vi "SoftwarePhase.vi"() -> ()   [LabVIEW 2012]
uses:
  <vilib>/imath/engines/lvmath/Plug In/_Char/NIMS_CH_character datatype.ctl
  <vilib>/Utility/inputDevices.llb/closeKeyboard.vi
  <vilib>/imath/engines/lvmath2/RunTimeEngine/ErrorHandling/NIMS_Finalize Error.vi
  <vilib>/imath/engines/lvmath2/RunTimeEngine/Managers/WorkSpace/UID Generator.vi
  <vilib>/imath/engines/lvmath2/RunTimeEngine/Managers/SymbolTable/Clear UID.vi
  <vilib>/imath/engines/lvmath/Plug In/_Char/NIMS_CH_Character RV to String.vi
  <vilib>/imath/engines/lvmath2/RunTimeEngine/NodeEndStatement/NIMS_NodeEndStatement_Output.vi
  <instcachedir>/0/NIMS_NodeEndStatement_Output_53EC0D466D134D7ABD903AC30B43404B.lvgen/NIMS_NodeEndStatement_Output_53EC0D466D134D7ABD903AC30B43404B_009.vi
  <vilib>/imath/engines/lvmath2/RunTimeEngine/RunTimeType/NIMS_RunTimeType_From StrictType (excl LVString).vi
  <instcachedir>/0/NIMS_RunTimeType_From StrictType (excl LVString)_AC52D965D0864706932D20A05968E122.lvgen/NIMS_RunTimeType_From StrictType (excl LVString)_AC52D965D0864706932D20A05968E122_001.vi
  <vilib>/imath/engines/lvmath2/RunTimeEngine/LocalVariableDefStatement/MC_LocalVariableDefStatement_Display.vi
  <vilib>/imath/engines/lvmath2/RunTimeEngine/VariableToken/NIMS_VariableToken_CondDefined.vi
  <instcachedir>/0/NIMS_VariableToken_CondDefined_295AAB8C64C949DA8EA45AB7820AF759.lvgen/NIMS_VariableToken_CondDefined_295AAB8C64C949DA8EA45AB7820AF759_004.vi
  <vilib>/imathl/engines/lvmath/Functions/Error Handling/Create Error.vi
  <instcachedir>/0/NIMS_NodeEndStatement_Output_53EC0D466D134D7ABD903AC30B43404B.lvgen/NIMS_NodeEndStatement_Output_53EC0D466D134D7ABD903AC30B43404B_012.vi
  <instcachedir>/0/NIMS_RunTimeType_From StrictType (excl LVString)_AC52D965D0864706932D20A05968E122.lvgen/NIMS_RunTimeType_From StrictType (excl LVString)_AC52D965D0864706932D20A05968E122_000.vi
  <vilib>/imath/engines/lvmath2/RunTimeEngine/RunTimeType/NIMS_RunTimeType_Set Source Original Bool.vi
  <vilib>/Utility/inputDevices.llb/keyboardAcquire.vi
  <instcachedir>/0/NIMS_NodeEndStatement_Output_53EC0D466D134D7ABD903AC30B43404B.lvgen/NIMS_NodeEndStatement_Output_53EC0D466D134D7ABD903AC30B43404B_010.vi
  <vilib>/imath/engines/lvmath2/RunTimeEngine/Managers/SymbolTable/NIMS_WorkSpace.lvlib
panel:
  out "Simulation UDP":bool
  out "BS Timed Out":bool
  out "Base Station":string
  in  "error in (no error)":errorcluster
  in  "Tab Control":T1(tab)
  out "Bump Sensor 2":bool
  out "Distance 2, CM":dbl
  out "IR Volts 2":dbl
  out "Red":dbl(knob) scale=0.0..100.0
  out "Green":dbl(knob) scale=0.0..100.0
  out "Blue":dbl(knob) scale=0.0..100.0
  out "Color Chosen":u32(colorbox)
  out "Bump Sensor 1":bool
  out "IR Volts 1":dbl
  out "Distance 1, CM":dbl
  in  "stop":bool
  out "Left Rudder":i32
  out "Right Rudder":i32
  in  "Rudders":i32(slide)=1500 scale=500.0..2500.0
  out "Port\nMotor":i32
  out "Starboard\nMotor":i32
  out "Port Speed":i32(knob) scale=1000.0..2000.0
  out "Starboard Speed":i32(knob) scale=1000.0..2000.0
  in  "Pan Camera":i32(slide)=1500 scale=500.0..2500.0
  out "Speed Balance":i32(knob) scale=-600.0..600.0
  out "Angle to Target":i32
  out "Distance to Target":i32
  out "IR 2":bool
  out "IR 1":bool
  out "Bump 2":bool
  out "Bump  1":bool
  out "Current Target":i32
  out "Obstacle Detected":bool
  out "Primitive Engaged":string
  out "Desired Heading":i32
  out "Target Y":i32
  out "Target X":i32
  out "Current Y":i32
  out "Current X":i32
  out "Current Heading":i32
  in  "Target Approaching":i32
  out "Target Locations":i32[][](array[numeric])
  in  "Step Size":i32=5
  in  "PC Status":i32=1
  out "String Received":string
  out "return count":u32
  out "bytes written":u32
  out "Blinky":bool
  in  "String":string="$CS1500P1500R1500L1500P1500H   1\n"
  in  "FULLSTOP":bool
  in  "VISA resource name":refnum<visa-resource-name>="COM7"
  # "ROBOT CONTROL VI\nSoftware Phase for Autonomy\n\nVPreston\n3/20/2014"
  # "Use this tab to make sure your sensors are happy and working properly."
  # "Motor Control"
  # "Direction of thrust"
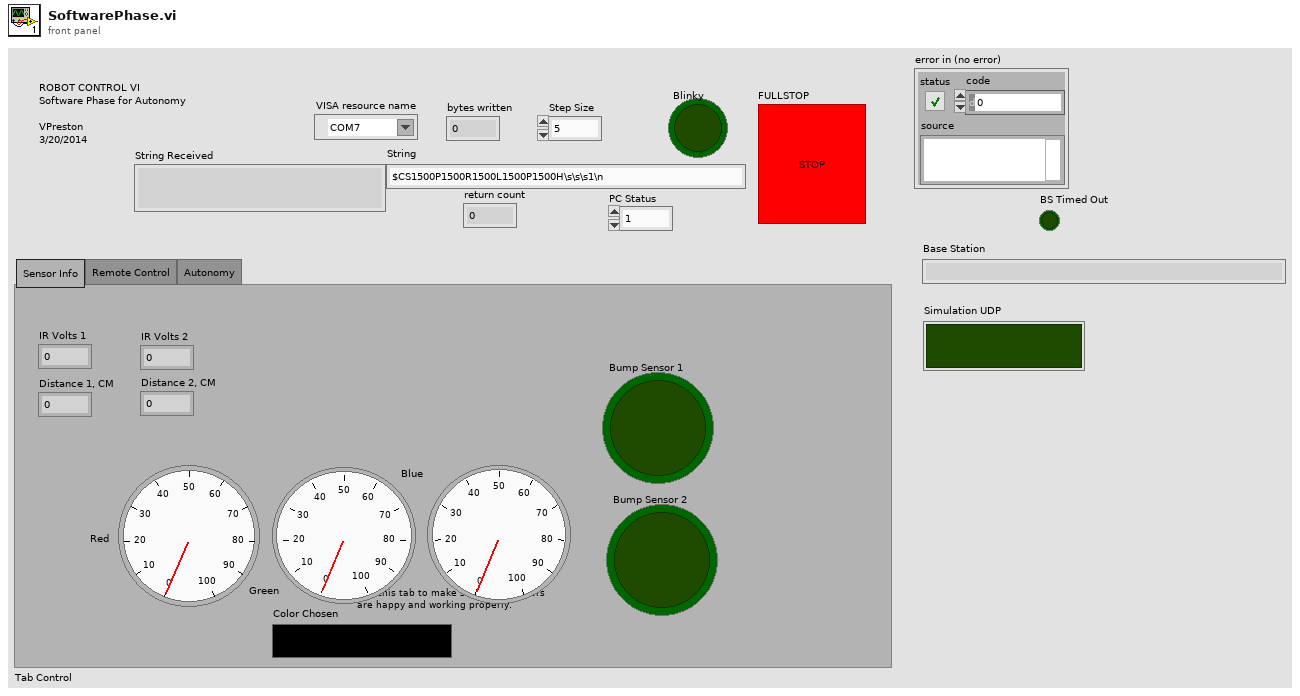
[diagram p1: front panel]
types:
  T1 = enum32{"Sensor Info", "Remote Control", "Autonomy"}
  T2 = enum16{"0", "1", "2", "3", "4", "5", "6", "7", "8", "9", "A", "B", "C", "D", "E", "F", "G", "H", "I", "J", "K", "L", "M", "N", "O", "P", "Q", "R", "S", "T", "U", "V", "W", "X", "Y", "Z", "F1", "F2", "F3", "F4", "F5", "F6", "F7", "F8", "F9", "F10", "F11", "F12", "F13", "F14", "F15", "ADD", "BACK", "BACKSLASH", "CAPITAL", "COMMA", "DECIMAL", "DELETE", "DIVIDE", "DOWN", "END", "EQUALS", "ESCAPE", "GRAVE (`)", "HOME", "INSERT", "LBRACKET", "LCONTROL", "LEFT", "L ALT", "LSHIFT", "LWIN", "MINUS", "MULTIPLY", "NEXT", "NUMLOCK", "NUMPAD_0", "NUMPAD_1", "NUMPAD_2", "NUMPAD_3", "NUMPAD_4", "NUMPAD_5", "NUMPAD_6", "NUMPAD_7", "NUMPAD_8", "NUMPAD_9", "PAUSE", "PERIOD", "PRIOR (PG UP)", "RBRACKET", "RCONTROL", "RETURN", "RIGHT", "R ALT", "RSHIFT", "RWIN", "SCROLL", "SEMICOLON", "SLASH", "SPACE", "SUBTRACT", "TAB", "UP", "ENTER (num pad)", "' (quote)"}[]
  T3 = enum16{"0", "1", "2", "3", "4", "5", "6", "7", "8", "9", "A", "B", "C", "D", "E", "F", "G", "H", "I", "J", "K", "L", "M", "N", "O", "P", "Q", "R", "S", "T", "U", "V", "W", "X", "Y", "Z", "F1", "F2", "F3", "F4", "F5", "F6", "F7", "F8", "F9", "F10", "F11", "F12", "F13", "F14", "F15", "ADD", "BACK", "BACKSLASH", "CAPITAL", "COMMA", "DECIMAL", "DELETE", "DIVIDE", "DOWN", "END", "EQUALS", "ESCAPE", "GRAVE (`)", "HOME", "INSERT", "LBRACKET", "LCONTROL", "LEFT", "L ALT", "LSHIFT", "LWIN", "MINUS", "MULTIPLY", "NEXT", "NUMLOCK", "NUMPAD_0", "NUMPAD_1", "NUMPAD_2", "NUMPAD_3", "NUMPAD_4", "NUMPAD_5", "NUMPAD_6", "NUMPAD_7", "NUMPAD_8", "NUMPAD_9", "PAUSE", "PERIOD", "PRIOR (PG UP)", "RBRACKET", "RCONTROL", "RETURN", "RIGHT", "R ALT", "RSHIFT", "RWIN", "SCROLL", "SEMICOLON", "SLASH", "SPACE", "SUBTRACT", "TAB", "UP", "ENTER (num pad)", "' (quote)"}
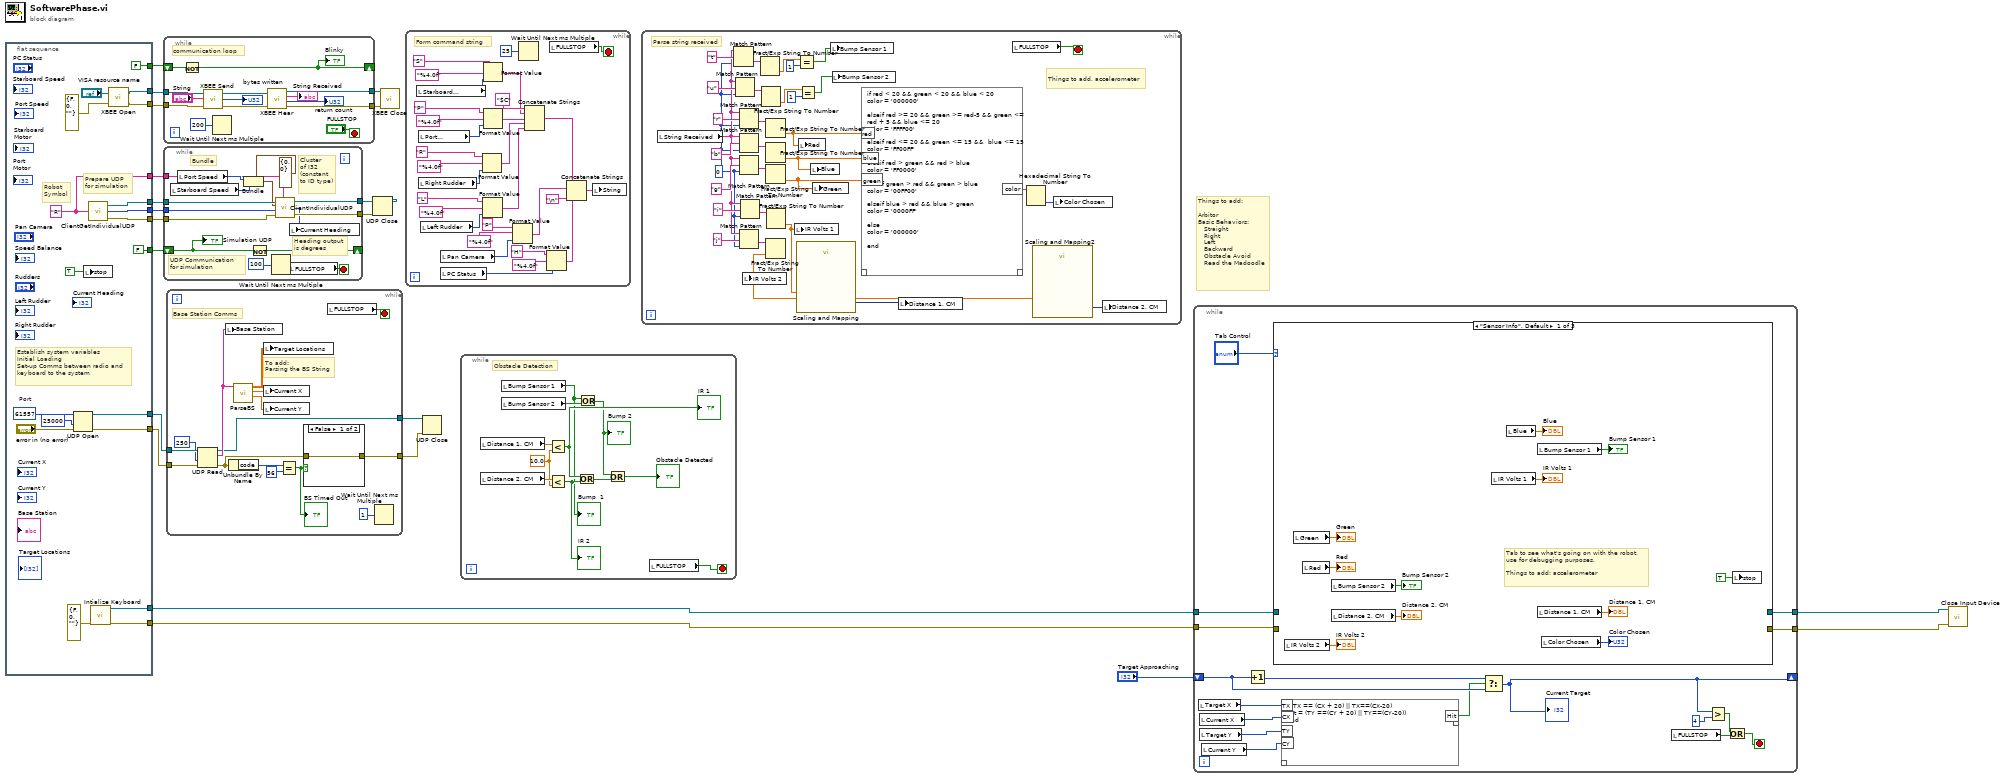
[diagram p0: block diagram]
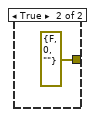
[diagram p2: hidden frame]
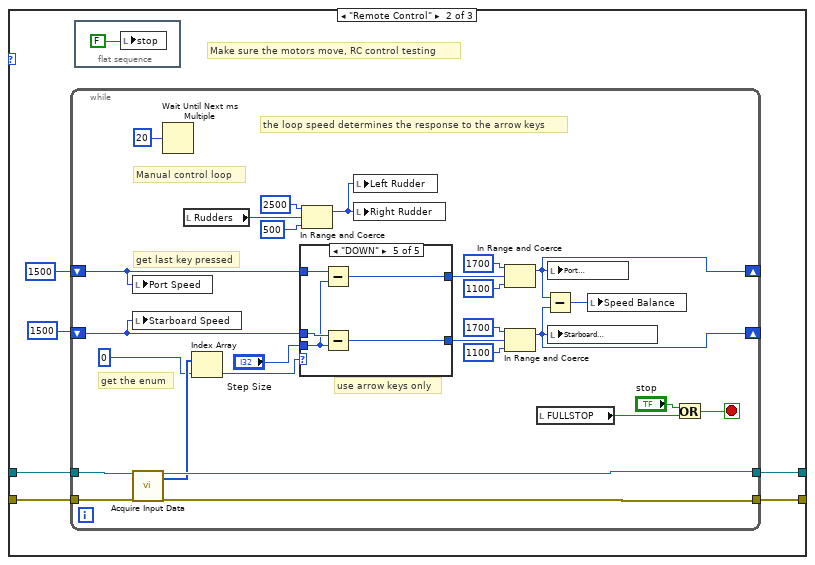
[diagram p3: hidden frame]
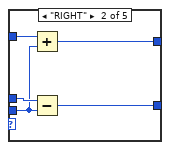
[diagram p5: hidden frame]
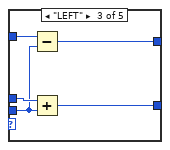
[diagram p6: hidden frame]
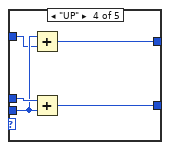
[diagram p7: hidden frame]
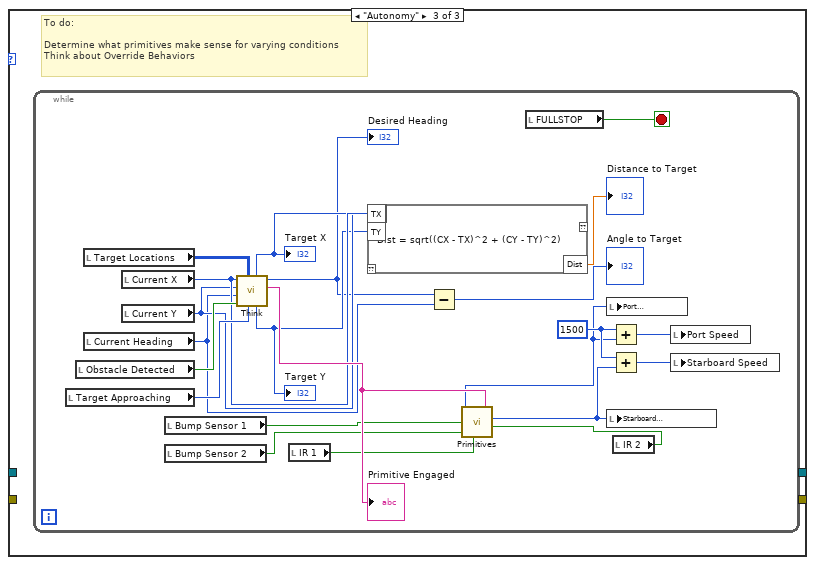
[diagram p8: hidden frame]
diagram:
  # "Things to add: \n\nArbitor\nBasic Behaviors:\n   Straight\n   Right\n   Left\n   Backward\n   Obstacle Avoid\n   Read the Madoodle"
  n1 = flat-sequence {
    tunnel: [w40] -> w21
    tunnel: [w23] -> w20
    tunnel: [FALSE] -> w17
    tunnel: [w35] -> w16
    tunnel: [w34] -> w15
    tunnel: [w29] -> w8
    tunnel: [w28] -> w12
    tunnel: [w27] -> w7
    tunnel: [w26] -> w5
    tunnel: [w25] -> w6
    tunnel: [w24] -> w4
    tunnel: [FALSE] -> w1
    frame #0 {
      w24 = "R"
      w31 = u16 61557  # Port
      # "Prepare UDP\nfor simulation"
      # "Robot \nSymbol"
      # "Establish system variables\nInitial Loading\nSet-up Comms between radio and\nkeyboard to the system"
      n2 = UDP Open(8:"error in (no error)", 9:25000 ("timeout ms (25000)"), 11:w31) -> (port=w29:refnum<k16>, 0:w28:errorcluster)  [unwired: 2 in, 1 out]
      n3 = local write "stop"(TRUE) -> ()
      n4 = call "ClientGetIndividualUDP.vi"("Robot Symbol"=w24) -> ("UDP Connection ID"=w27:refnum<k16>, "Remote Port #"=w26:i32, "error out"=w25:errorcluster)
      n5 = call <vilib>:"Intialize Keyboard.vi"("error in (no error)"=errorcluster {"status"=FALSE, "code"=0, "source"=""}) -> ("error out"=w34:errorcluster, "device ID"=w35:refnum<k1>)  [unwired: 9 in]
      n6 = call "XBEE Open.vi"("error in"=errorcluster {"status"=FALSE, "code"=0, "source"=""}, "VISA resource name"="VISA resource name") -> ("error out"=w23:errorcluster, "VISA resource name out"=w40:refnum<visa-resource-name>)
    }
  }
  n7 = while {
    tunnel: w21 -> [w53]
    tunnel: w20 -> [w52]
    tunnel: [w47] -> w19
    tunnel: [w46] -> w18
    shift-right: [w50] -> _
    shift-left: w17 -> [w51]
    stop <- "FULLSTOP" stop-if-true
    # "communication loop"
    n8 = Not(x=w51) -> (.not. x?=w50:bool)
    "Blinky" <- w50
    n9 = call "XBEE Send.vi"("error in (no error)"=w52, "String"="String", "VISA resource name"=w53) -> ("error out"=w43:errorcluster, "return count"=→"bytes written":u32, "VISA resource name out"=w44:refnum<visa-resource-name>)
    n10 = Wait Until Next ms Multiple(millisecond multiple=u32 200) -> ()  [unwired: 1 out]
    n11 = call "XBEE Hear.vi"("VISA resource name"=w44, "error in (no error)"=w43) -> ("VISA resource name out"=w47:refnum<visa-resource-name>, "String Received"=→"String Received":string, "return count"=→"return count":u32, "error out"=w46:errorcluster)
  }
  n12 = while {
    tunnel: w6 -> [w56]
    tunnel: w7 -> [w69]
    tunnel: w5 -> [w68]
    tunnel: [w63] -> w3
    tunnel: [w62] -> w2
    shift-right: [w59] -> _
    shift-left: w1 -> [w58]
    tunnel: w4 -> [w55]
    stop <- w60 stop-if-true
    # "UDP Communication \nfor simulation"
    # "Heading output\nis degrees"
    # "Cluster\nof I32\n(constant\nto ID type)"
    # "Bundle"
    n13 = local read "Starboard Speed"() -> (w66:i32)
    n14 = local read "Port Speed"() -> (w67:i32)
    n15 = Bundle(cluster=cluster{i32, i32} {0, 0}, w67, w66) -> (w65:cluster{i32, i32})
    n16 = Not(x=w58) -> (.not. x?=w59:bool)
    n17 = Wait Until Next ms Multiple(millisecond multiple=u32 100) -> ()  [unwired: 1 out]
    n18 = call "ClientIndividualUDP.vi"("UDP Connection ID"=w69, "Rover Inputs"=w65, "Remote Port #"=w68, "error in (no error)"=w56, "Robot Symbol"=w55) -> ("connection ID out"=w63:refnum<k16>, "Robot Heading"=w61:i32, "error out"=w62:errorcluster)
    n19 = local read "FULLSTOP"() -> (w60:bool)
    n20 = local write "Current Heading"(w61) -> ()
    "Simulation UDP" <- w58
  }
  n21 = while {
    tunnel: w8 -> [w84]
    tunnel: w12 -> [w83]
    tunnel: [w71] -> w10
    tunnel: [w70] -> w9
    stop <- w76 stop-if-true
    # "To add: \nParsing the BS String"
    # "Base Station Comms"
    n22 = UDP Read(connection ID=w84, timeout ms (25000)=250, 8:w83) -> (data out=w75:string, error out=w79:errorcluster, 3:w71:refnum<k16>)  [unwired: 1 in, 2 out]
    n23 = local write "Base Station"(w75) -> ()
    n24 = Unbundle By Name(w79) -> ("code"=w78:i32)
    n25 = call "ParseBS.vi"("BS String"=w75) -> ("Y Pos"=w72:dbl, "X Pos"=w73:dbl, "Target Locations"=w74:dbl[][])  [unwired: 8 in]
    n26 = local write "Target Locations"(w74) -> ()
    n27 = local write "Current X"(w73) -> ()
    n28 = local write "Current Y"(w72) -> ()
    n29 = Equal?(x=w78, y=56) -> (x = y?=w77:bool)
    "BS Timed Out" <- w77
    n30 = case shown="False" w77 {
      tunnel: [w85 errorcluster {"status"=FALSE, "code"=0, "source"=""} ("error out")] -> w70
      tunnel: w79 -> [w85 _]
      frame False {
      }
      frame True {
      }
    }
    n31 = local read "FULLSTOP"() -> (w76:bool)
    n32 = Wait Until Next ms Multiple(millisecond multiple=u32 1) -> ()  [unwired: 1 out]
  }
  n33 = UDP Close(connection ID=w3, 8:w2) -> ()  [unwired: 2 out]
  n34 = call "XBEE Close.vi"("error in (no error)"=w18, "VISA resource name"=w19) -> ()
  n35 = while {
    stop <- w116 stop-if-true
    # "Form command string"
    n36 = local read "Starboard\nMotor"() -> (w113:i32)
    n37 = local read "Port\nMotor"() -> (w110:i32)
    n38 = local read "Right Rudder"() -> (w104:i32)
    n39 = local read "Left Rudder"() -> (w101:i32)
    n40 = local read "Pan Camera"() -> (w95:i32)
    n41 = local read "PC Status"() -> (w92:i32)
    n42 = Format Value(string ("")="R", format string="%4.0f", value (0)=w104) -> (output string=w100:string)
    n43 = Format Value(string ("")="L", format string="%4.0f", value (0)=w101) -> (output string=w99:string)
    n44 = Format Value(string ("")="S", format string="%4.0f", value (0)=w113) -> (output string=w108:string)
    n45 = Format Value(string ("")="P", format string="%4.0f", value (0)=w110) -> (output string=w107:string)
    n46 = Format Value(string ("")="P", format string="%4.0f", value (0)=w95) -> (output string=w90:string)
    n47 = Wait Until Next ms Multiple(millisecond multiple=u32 25) -> ()  [unwired: 1 out]
    n48 = Concatenate Strings("$C", w108, w107, w100, w99) -> (w91:string)
    n49 = Format Value(string ("")="H", format string="%4.0f", value (0)=w92) -> (output string=w89:string)
    n50 = local read "FULLSTOP"() -> (w116:bool)
    n51 = Concatenate Strings(w91, w90, w89, "\n") -> (w96:string)
    n52 = local write "String"(w96) -> ()
  }
  n53 = UDP Close(connection ID=w10, 8:w9) -> ()  [unwired: 2 out]
  n54 = while {
    stop <- w127 stop-if-true
    w123 = 10.0 ("y")
    # "Obstacle Detection"
    n55 = local read "Distance 1, CM"() -> (w125:dbl)
    n56 = local read "Distance 2, CM"() -> (w124:dbl)
    n57 = local read "Bump Sensor 1"() -> (w118:bool)
    "Bump  1" <- w118
    n58 = local read "Bump Sensor 2"() -> (w126:bool)
    n59 = Less?(x=w125, y=w123) -> (x < y?=w119:bool)
    "IR 1" <- w119
    n60 = Less?(x=w124, y=w123) -> (x < y?=w120:bool)
    "IR 2" <- w120
    n61 = Or(x=w119, y=w120) -> (x .or. y?=w122:bool)
    n62 = Or(x=w118, y=w126) -> (x .or. y?=w117:bool)
    "Bump 2" <- w117
    n63 = Or(x=w117, y=w122) -> (x .or. y?=→"Obstacle Detected":bool)
    n64 = local read "FULLSTOP"() -> (w127:bool)
  }
  n65 = while {
    stop <- w159 stop-if-true
    w129 = 0 ("offset (0)")
    # "Things to add, accelerometer"
    # "Parse string received"
    n66 = local read "String Received"() -> (w130:string)
    n67 = Match Pattern(string=w130, regular expression="t", offset (0)=w129) -> (after substring=w146:string)  [unwired: 3 out]
    n68 = Match Pattern(string=w130, regular expression="u", offset (0)=w129) -> (after substring=w131:string)  [unwired: 3 out]
    n69 = Match Pattern(string=w130, regular expression="r", offset (0)=w129) -> (after substring=w149:string)  [unwired: 3 out]
    n70 = Match Pattern(string=w130, regular expression="b", offset (0)=w129) -> (after substring=w147:string)  [unwired: 3 out]
    n71 = Match Pattern(string=w130, regular expression="g", offset (0)=w129) -> (after substring=w148:string)  [unwired: 3 out]
    n72 = Match Pattern(string=w130, regular expression="j", offset (0)=w129) -> (after substring=w137:string)  [unwired: 3 out]
    n73 = Match Pattern(string=w130, regular expression="i", offset (0)=w129) -> (after substring=w150:string)  [unwired: 3 out]
    n74 = Fract/Exp String To Number(string=w146) -> (number=w157:dbl)  [unwired: 3 in, 1 out]
    n75 = Fract/Exp String To Number(string=w131) -> (number=w134:dbl)  [unwired: 3 in, 1 out]
    n76 = Fract/Exp String To Number(string=w149) -> (number=w143:dbl)  [unwired: 3 in, 1 out]
    n77 = Fract/Exp String To Number(string=w147) -> (number=w142:dbl)  [unwired: 3 in, 1 out]
    n78 = Fract/Exp String To Number(string=w148) -> (number=w141:dbl)  [unwired: 3 in, 1 out]
    n79 = Fract/Exp String To Number(string=w137) -> (number=w136:dbl)  [unwired: 3 in, 1 out]
    n80 = local write "IR Volts 2"(w136) -> ()
    n81 = Fract/Exp String To Number(string=w150) -> (number=w140:dbl)  [unwired: 3 in, 1 out]
    n82 = local write "IR Volts 1"(w140) -> ()
    n83 = call "Scaling and Mapping"("Signals"=w140) -> ("Scaled Signals"=w139:dynamicdata)  [unwired: 9 in, 1 out]
    n84 = Equal?(x=w157, y=1) -> (x = y?=w144:bool)
    n85 = Equal?(x=w134, y=1) -> (x = y?=w128:bool)
    n86 = local write "Red"(w143) -> ()
    n87 = local write "Blue"(w142) -> ()
    n88 = local write "Green"(w141) -> ()
    n89 = local write "Bump Sensor 1"(w144) -> ()
    n90 = local write "Bump Sensor 2"(w128) -> ()
    n91 = mathscript code="if red < 20 && green < 20 && blue < 20\ncolor = '000000'\n\nelseif red >= 20 && green >= red-5 && green <= red + 5 && blue <= 20\ncolor = 'FFFF00'\n\nelseif red <= 20 && green <= 15 &&  blue <= 15\ncolor = 'FF00FF'\n\nelseif red > green && red > blue\ncolor = 'FF0000'\n\nelseif green > red && green > blue\ncolor = '00FF00'\n\nelseif blue > red && blue > green\ncolor = '0000FF' \n\nelse\ncolor = '000000'\n\nend"("red"=w143, "blue"=w142, "green"=w141) -> ("color"=w158:string)  [unwired: 1 in, 1 out]
    n92 = local write "Distance 1, CM"(w139) -> ()
    n93 = local read "FULLSTOP"() -> (w159:bool)
    n94 = Hexadecimal String To Number(string=w158) -> (number=w145:u32)  [unwired: 2 in, 1 out]
    n95 = call "Scaling and Mapping2"("Signals"=w136) -> ("Scaled Signals"=w135:dynamicdata)  [unwired: 9 in, 1 out]
    n96 = local write "Color Chosen"(w145) -> ()
    n97 = local write "Distance 2, CM"(w135) -> ()
  }
  n98 = while {
    tunnel: w16 -> [w461]
    tunnel: w15 -> [w460]
    tunnel: [w459] -> w14
    tunnel: [w458] -> w13
    shift-right: [w451] -> _
    shift-left: "Target Approaching" -> [w456]
    stop <- w454 stop-if-true
    n99 = local read "Target X"() -> (w450:i32)
    n100 = local read "Current X"() -> (w449:i32)
    n101 = local read "Target Y"() -> (w448:i32)
    n102 = local read "Current Y"() -> (w447:i32)
    n103 = Increment(x=w456) -> (x+1=w457:i32)
    n104 = case shown="\"Sensor Info\", Default" "Tab Control" {
      tunnel: w461 -> [_ w566 _]
      tunnel: w460 -> [_ w565 _]
      tunnel: [_ w562 _] -> w459
      tunnel: [_ w561 _] -> w458
      frame "Sensor Info", Default {
        # "Tab to see what's going on with the robot, \nuse for debugging purposes.  \n\nThings to add: accelerometer"
        n105 = local read "IR Volts 2"() -> (→"IR Volts 2":dbl)
        n106 = local read "Green"() -> (→"Green":dbl)
        n107 = local read "Red"() -> (→"Red":dbl)
        n108 = local read "Bump Sensor 2"() -> (→"Bump Sensor 2":bool)
        n109 = local read "Distance 2, CM"() -> (→"Distance 2, CM":dbl)
        n110 = local read "IR Volts 1"() -> (→"IR Volts 1":dbl)
        n111 = local read "Blue"() -> (→"Blue":dbl)
        n112 = local read "Bump Sensor 1"() -> (→"Bump Sensor 1":bool)
        n113 = local read "Distance 1, CM"() -> (→"Distance 1, CM":dbl)
        n114 = local read "Color Chosen"() -> (→"Color Chosen":u32)
        n115 = local write "stop"(TRUE) -> ()
      }
      frame "Remote Control" {
        # "Make sure the motors move, RC control testing"
        n116 = while {
          tunnel: [w594] -> w561
          tunnel: [w593] -> w562
          shift-right: [w577] -> _
          shift-left: 1500 -> [w579]
          shift-right: [w576] -> _
          shift-left: 1500 -> [w578]
          tunnel: w566 -> [w569]
          tunnel: w565 -> [w568]
          stop <- w570 stop-if-true
          # "use arrow keys only"
          # "Manual control loop"
          # "get the enum"
          # "the loop speed determines the response to the arrow keys"
          # "get last key pressed"
          n117 = local write "Port Speed"(w578) -> ()
          n118 = local write "Starboard Speed"(w579) -> ()
          n119 = call-poly <vilib>:"Acquire Input Data.vi"("device ID"=w569, "error in (no error)"=w568) -> ("device ID"=w593:refnum<k1>, "keys pressed"=w592:T2, "error out"=w594:errorcluster)  [unwired: 15 in]
          n120 = Wait Until Next ms Multiple(millisecond multiple=u32 20) -> ()  [unwired: 1 out]
          n121 = local read "Rudders"() -> (w574:i32)
          n122 = Index Array(array=w592, index=0) -> (element=w590:T3)
          n123 = case shown="\"DOWN\"" w590 {
            tunnel: w579 -> [w596 w598 w603 w611 w616]
            tunnel: [w596 w599 w604 w610 w615] -> w588
            tunnel: w578 -> [w595 w601 w605 w608 w614]
            tunnel: [w595 w600 w606 w607 w612] -> w580
            tunnel: "Step Size" -> [_ w597 w602 w609 w613]
            frame "0", Default {
            }
            frame "RIGHT" {
              n124 = Add(x=w601, y=w597) -> (x+y=w600:i32)
              n125 = Subtract(x=w598, y=w597) -> (x-y=w599:i32)
            }
            frame "LEFT" {
              n126 = Subtract(x=w605, y=w602) -> (x-y=w606:i32)
              n127 = Add(x=w603, y=w602) -> (x+y=w604:i32)
            }
            frame "UP" {
              n128 = Add(x=w609, y=w608) -> (x+y=w607:i32)
              n129 = Add(x=w611, y=w609) -> (x+y=w610:i32)
            }
            frame "DOWN" {
              n130 = Subtract(x=w614, y=w613) -> (x-y=w612:i32)
              n131 = Subtract(x=w616, y=w613) -> (x-y=w615:i32)
            }
          }
          n132 = In Range and Coerce(upper limit=2500, x=w574, lower limit=500) -> (coerced(x)=w573:i32)  [unwired: 1 out]
          n133 = local write "Left Rudder"(w573) -> ()
          n134 = local write "Right Rudder"(w573) -> ()
          n135 = In Range and Coerce(upper limit=1700, x=w580, lower limit=1100) -> (coerced(x)=w576:i32)  [unwired: 1 out]
          n136 = In Range and Coerce(upper limit=1700, x=w588, lower limit=1100) -> (coerced(x)=w577:i32)  [unwired: 1 out]
          n137 = local read "FULLSTOP"() -> (w571:bool)
          n138 = Subtract(x=w576, y=w577) -> (x-y=w575:i32)
          n139 = local write "Port\nMotor"(w576) -> ()
          n140 = local write "Starboard\nMotor"(w577) -> ()
          n141 = local write "Speed Balance"(w575) -> ()
          n142 = Or(x="stop", y=w571) -> (x .or. y?=w570:bool)
        }
        n143 = flat-sequence {
          frame #0 {
            n144 = local write "stop"(FALSE) -> ()
          }
        }
      }
      frame "Autonomy" {
        # "To do:\n\nDetermine what primitives make sense for varying conditions\nThink about Override Behaviors"
        n145 = while {
          stop <- w617 stop-if-true
          w620 = 1500
          n146 = local read "Target Approaching"() -> (w636:i32)
          n147 = local read "Obstacle Detected"() -> (w637:bool)
          n148 = local read "Target Locations"() -> (w638:i32[][])
          n149 = local read "Current Heading"() -> (w624:i32)
          n150 = local read "Current X"() -> (w630:i32)
          n151 = local read "Current Y"() -> (w629:i32)
          n152 = local read "Bump Sensor 1"() -> (w634:bool)
          n153 = local read "Bump Sensor 2"() -> (w633:bool)
          n154 = call "Think.vi"("Target"=w636, "Target Locations"=w638, "Override Engaged"=w637, "Current Heading"=w624, "Y Position"=w629, "X Position"=w630) -> ("Executable Primitive"=w635:string, "Desired Heading"=w625:i32, "Desired Y"=w627:i32, "Desired X"=w628:i32)  [unwired: 2 in]
          "Target Y" <- w627
          "Desired Heading" <- w625
          "Primitive Engaged" <- w635
          "Target X" <- w628
          n155 = local read "IR 1"() -> (w632:bool)
          n156 = mathscript code="Dist = sqrt((CX - TX)^2 + (CY - TY)^2)"("CX"=w630, "CY"=w629, "TX"=w628, "TY"=w627) -> ("Dist"=→"Distance to Target":cdb)  [unwired: 1 in, 1 out]
          n157 = Subtract(x=w625, y=w624) -> (x-y=→"Angle to Target":i32)
          n158 = local read "FULLSTOP"() -> (w617:bool)
          n159 = local read "IR 2"() -> (w631:bool)
          n160 = call "Primitives.vi"("Bump 1"=w634, "Bump 2"=w633, "IR 1"=w632, "Primitive"=w635, "IR 2"=w631) -> ("Port Speed"=w619:i32, "Starboard Speed"=w622:i32)  [unwired: 2 in]
          n161 = local write "Port\nMotor"(w619) -> ()
          n162 = local write "Starboard\nMotor"(w622) -> ()
          n163 = Add(x=w620, y=w619) -> (x+y=w618:i32)
          n164 = Add(x=w620, y=w622) -> (x+y=w621:i32)
          n165 = local write "Port Speed"(w618) -> ()
          n166 = local write "Starboard Speed"(w621) -> ()
        }
      }
    }
    n167 = mathscript code="if TX == (CX + 20) || TX==(CX-20)\nHit = (TY ==(CY + 20) || TY==(CY-20))\nend"("TX"=w450, "TY"=w448, "CX"=w449, "CY"=w447) -> ("Hit"=w446:bool)  [unwired: 1 in, 1 out]
    n168 = Select(t=w457, s=w446, f=w456) -> (s? t:f=w451:i32)
    "Current Target" <- w451
    n169 = local read "FULLSTOP"() -> (w455:bool)
    n170 = Greater?(x=w451, y=4) -> (0:w452:bool)
    n171 = Or(x=w452, y=w455) -> (x .or. y?=w454:bool)
  }
  n172 = call-poly <vilib>:"Close Input Device.vi"("error in (no error)"=w13, "device ID"=w14) -> ()  [unwired: 8 in, 1 out]
